vi "Delete Channels From End.vi"(8 "Channel Label":string, 9 "Prior Number of Channels":i32, 10 "Number of Channels to Delete":i32, 11 "UI Data in":refnum<class "Settings UI.lvclass">) -> (3 "UI Data out":refnum<class "Settings UI.lvclass">)   [LabVIEW 2024, in "Output Sequencer.lvlib" / "Settings UI.lvclass"]
uses:
  Settings UI.lvclass
  Settings UI.lvclass/Settings UI.ctl
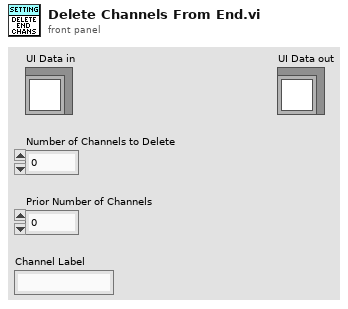
[diagram p1: front panel]
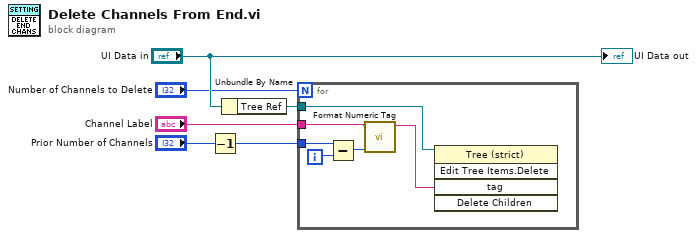
[diagram p0: block diagram]
diagram:
  n1 = Decrement(x="Prior Number of Channels") -> (x-1=w1:i32)
  n2 = Unbundle By Name("UI Data in") -> ("Tree Ref"=w3:refnum<vi>)
  n3 = for {
    N: "Number of Channels to Delete" -> [_]
    tunnel: w1 -> [w12]
    tunnel: "Channel Label" -> [w9]
    tunnel: w3 -> [w10]
    i -> [w11]
    n4 = Subtract(x=w12, y=w11) -> (x-y=w7:i32)
    n5 = call "Format Numeric Tag.vi"("Number"=w7, "Tree label"=w9) -> ("Tag"=w8:string)  [unwired: 9 in]
    n6 = invoke class="Tree (strict)" method="Edit Tree Items.Delete"(reference=w10, "tag"=w8) -> ()  [unwired: 3 in, 5 out]
  }
  "UI Data out" <- "UI Data in"
